vi "Simple Single Point Benchmark.vi"() -> ()   [LabVIEW 2011]
uses:
  <instrlib>/niDMM/nidmm.llb/niDMM Function.ctl
  <instrlib>/niDMM/nidmm.llb/niDMM Auto Zero.ctl
  <instrlib>/niDMM/nidmm.llb/niDMM ADC Calibration.ctl
panel:
  in  "Resolution":dbl=1e-05 format="%.5f"
  out "Measurement Period (seconds)":dbl format="%.4f"
  in  "ADC Calibration":T1=-1 items=["Auto"=-1, "Off"=0, "On"=1]
  in  "Auto Zero":T2=1 items=["Auto"=-1, "Off"=0, "On"=1, "Once"=2]
  in  "Range":dbl=10.0 format="%.2f"
  in  "Function":T3
  in  "Instrument Descriptor":refnum<k15>="DMM"
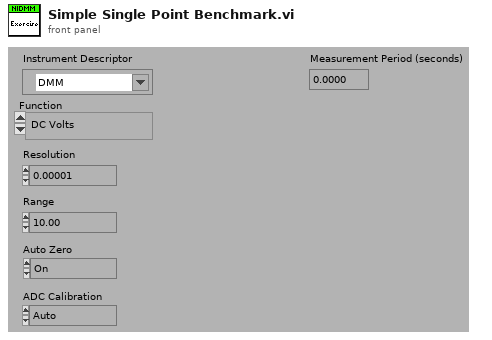
[diagram p1: front panel]
types:
  T1 = typedef "niDMM ADC Calibration.ctl" = i32
  T2 = typedef "niDMM Auto Zero.ctl" = i32
  T3 = typedef "niDMM Function.ctl" = enum16{"DC Volts", "AC Volts", "DC Current", "AC Current", "2-wire Resistance", "4-wire Resistance", "Diode", "Frequency", "Period", "AC Volts DC Coupled", "Capacitance", "Inductance", "Temperature"}
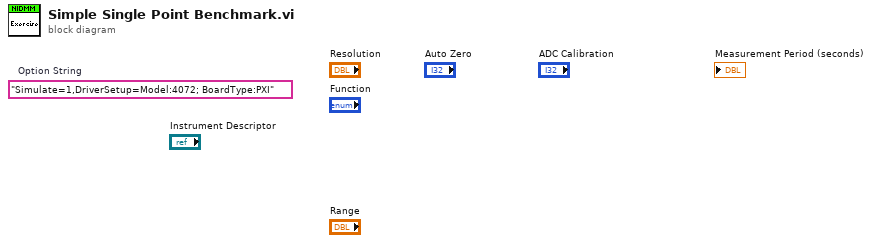
[diagram p0: block diagram]
diagram:
  (unwired) "Simulate=1,DriverSetup=Model:4072; BoardType:PXI"  # Option String
